vi "Write Path.vi"(8 "Error In":errorcluster, 10 "Pair":cluster{"Key":string, "Value":path}, 11 "Data In":refnum<class "Data.lvclass">) -> (0 "Error Out":errorcluster, 3 "Data Out":refnum<class "Data.lvclass">)   [LabVIEW 2018, in "Toolkit.lvlib" / "Loaders.lvlib" / "Data.lvclass"]
uses:
  Data.lvclass
  Data.lvclass/Data.ctl
  Data/Path/Path.lvclass
  D:/Users/cfield/Code/Field R&D Services/Mustache/LabVIEW/trunk/src/Toolkit/Data/Abstract/Abstract.lvclass
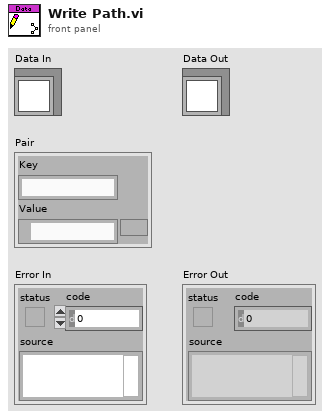
[diagram p1: front panel]
types:
  T1 = cluster{"Key":string, "Value":refnum<class "Abstract.lvclass">}[]
  T2 = cluster{"Key":string, "Path":refnum<class "Path.lvclass">}
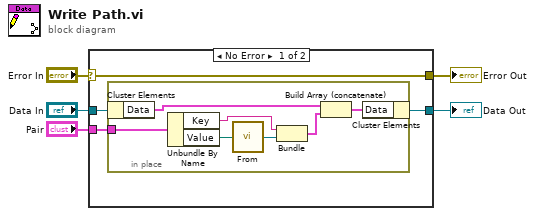
[diagram p0: block diagram]
diagram:
  n1 = case shown="No Error" "Error In" {
    selector: "Error In" -> [w9 w18]
    tunnel: [w9 w18] -> w4
    tunnel: [w7 w17] -> w2
    tunnel: "Data In" -> [w8 w17]
    tunnel: "Pair" -> [w6 _]
    frame No Error {
      n2 = in-place {
        in-place-border: w6 -> [w14]
        n3 = in-place-cluster #1(w8) -> ("Data"=w16:T1)
        n4 = Unbundle By Name(w14) -> ("Key"=w12:string, "Value"=w13:path)
        n5 = call "From.vi"("Value"=w13) -> ("Path"=w11:refnum<class "Path.lvclass">)
        n6 = Bundle("Key"=w12, "Path"=w11) -> (w10:T2)  [unwired: 1 in]
        n7 = Build Array (concatenate)(w16, w10) -> (w15:T1)
        n8 = in-place-cluster #1("Data"=w15) -> (w7:refnum<class "Data.lvclass">)
      }
    }
    frame Error {
    }
  }
  "Error Out" <- w4
  "Data Out" <- w2
